vi "Cleanup Events.vi"(8 "error in (no error)":errorcluster, 11 "Events":T1) -> ()   [LabVIEW 2020, in "TSS.lvlib" / "Engine.lvclass"]
uses:
  Engine.lvclass
  Events.ctl
  Create VC Event Data.ctl
  Variable Container Type.ctl
  VariableContainer/Typedefs/Session Handle.ctl
  VariableContainer/VariableContainer.lvclass
  Create Report Event Data.ctl
  Execution/Typedefs/Session Handle.ctl
  Execution/Execution.lvclass
  Report/Typedefs/Session Handle.ctl
  Report/Report.lvclass
  Open Sequence File Event Data.ctl
  Data Types/File Load Options.ctl
  SequenceFile/Typedefs/Session Handle.ctl
  SequenceFile/SequenceFile.lvclass
  Session Notification.ctl
  Prepare Execution Event Data.ctl
  Execution/Execution Options.ctl
  TSS.lvlib
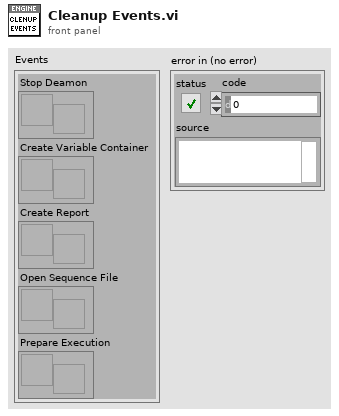
[diagram p1: front panel]
types:
  T1 = typedef "TSS.lvlib/Engine.lvclass/Events.ctl" = cluster{"Stop Deamon":refnum<user-event>, "Create Variable Container":refnum<user-event>, "Create Report":refnum<user-event>, "Open Sequence File":refnum<user-event>, "Prepare Execution":refnum<user-event>}
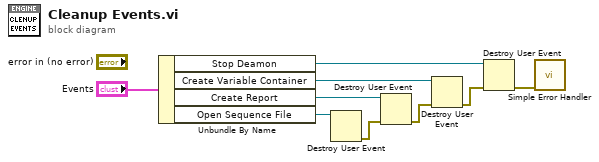
[diagram p0: block diagram]
diagram:
  n1 = Unbundle By Name("Events") -> ("Stop Deamon"=w9:refnum<user-event>, "Create Variable Container"=w8:refnum<user-event>, "Create Report"=w7:refnum<user-event>, "Open Sequence File"=w5:refnum<user-event>)
  n2 = Destroy User Event(user event=w5) -> (error out=w4:errorcluster)  [unwired: 1 in]
  n3 = Destroy User Event(user event=w7, error in=w4) -> (error out=w3:errorcluster)
  n4 = Destroy User Event(user event=w8, error in=w3) -> (error out=w2:errorcluster)
  n5 = Destroy User Event(user event=w9, error in=w2) -> (error out=w1:errorcluster)
  n6 = call <vilib>:"Simple Error Handler.vi"("error in (no error)"=w1) -> ()  [unwired: 4 in, 5 out]
